vi "Script Accessors.vi"(4 "Project Ref":refnum<vi>, 5 "Type Path Map":map{path, path}(c390), 6 "Names":string[](array[string]), 7 "LVClass":refnum<vi>, 8 "error in (no error)":errorcluster, 10 "Updated Definition":refnum<class "Type.lvclass">[](array[class]), 11 "Accessors":T1[](array[typedef])) -> (0 "error":errorcluster)   [LabVIEW 2020, in "Conditum-Tools.lvlib" / "Entity Editor.lvclass"]
uses:
  Entity Editor.lvclass
  Conditum-Clone/Columns/Type/Type.lvclass
  Accessors.ctl
  Accessor Scope.ctl
  Conditum-Tools.lvlib
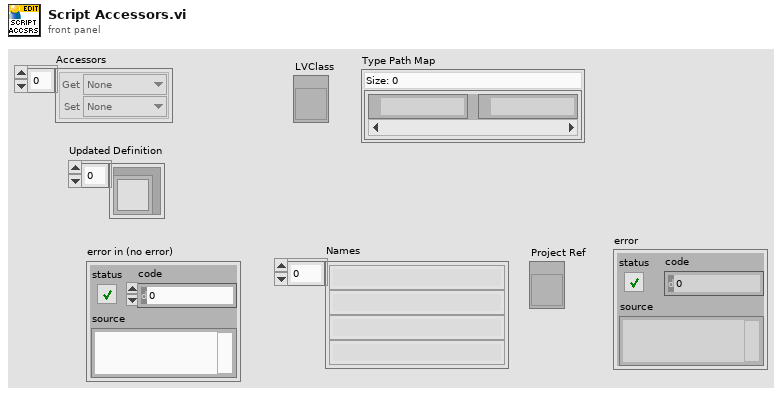
[diagram p1: front panel]
types:
  T1 = typedef "Conditum-Tools.lvlib/Accessors.ctl" = cluster{"Get":T2, "Set":T2}
  T2 = typedef "Conditum-Tools.lvlib/Accessor Scope.ctl" = enum16{"None", "Public", "Protected", "Private"}
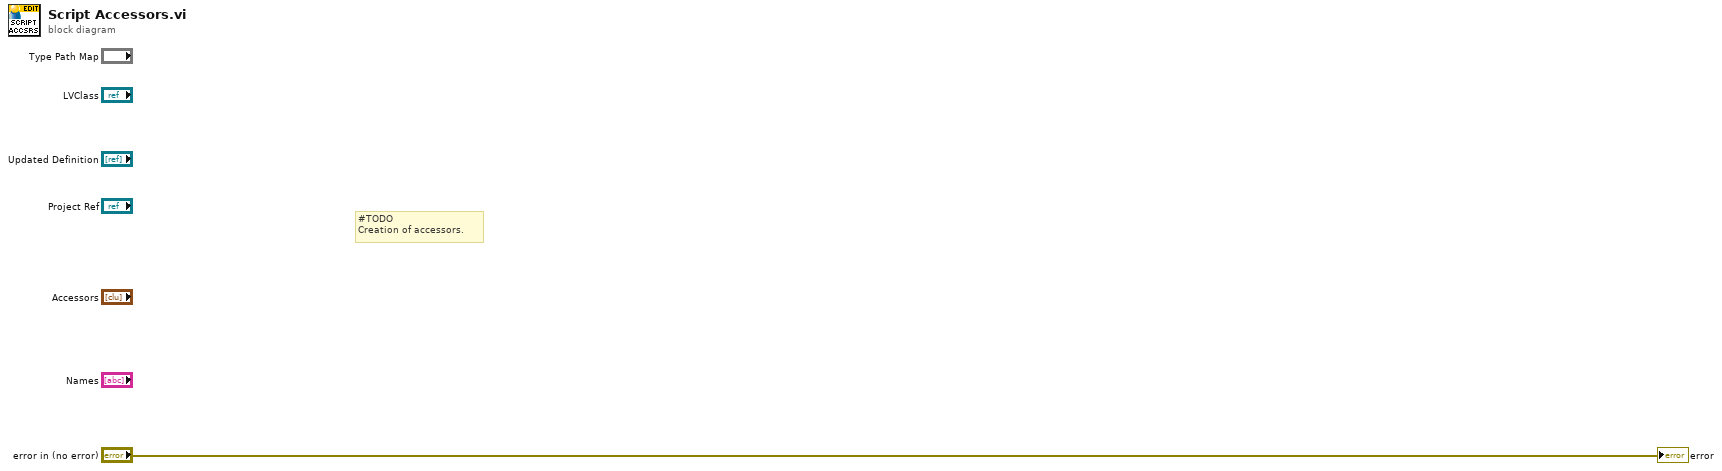
[diagram p0: block diagram]
diagram:
  # "#TODO\nCreation of accessors."
  "error" <- "error in (no error)"
